vi "Test HRTF Computation.vi"() -> ()   [LabVIEW 2015]
uses:
  Typedefs/HRTF-Window.ctl
  Typedefs/HRTF-Window Type.ctl
  <vilib>/Analysis/2dsp.llb/Real FFT.vi
  <vilib>/Analysis/2dsp.llb/Inverse Real FFT.vi
  <vilib>/Analysis/2dsp.llb/Rational Resample (single channel, DBL).vi
  Utility VIs/Conversion VIs/Create Waveform Cluster (1D).vi
  <vilib>/Analysis/NI_AALPro.lvlib
panel:
  in  "Window":T1={"Type"=enum."Hanning", "Length (ms)"=6.0, "Center (ms)"=5.0}
  out "Waveform Graph":cluster{dbl, "dx":dbl, "Y":dbl[]}(graph)
  in  "Path":path=path "D:/Data/HRTF/E02/work/Ear-elev0-az-60_L.txt"
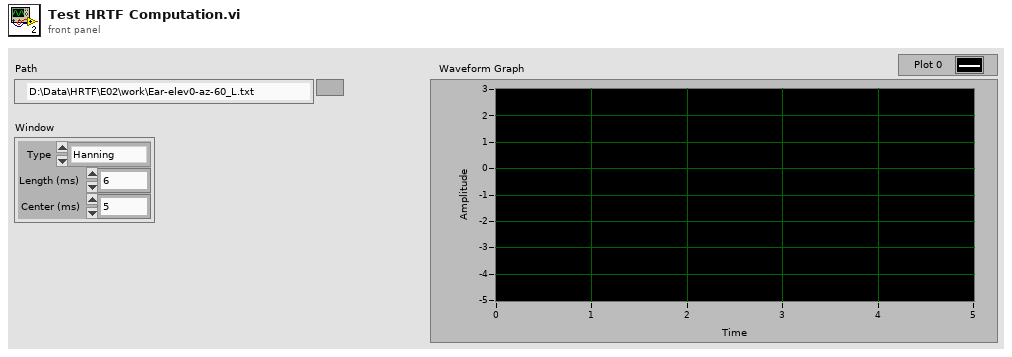
[diagram p1: front panel]
types:
  T1 = typedef "HRTF-Window.ctl" = cluster{"Type":T2, "Length (ms)":dbl, "Center (ms)":dbl}
  T2 = typedef "HRTF-Window Type.ctl" = enum16{"None", "Hanning"}
  T3 = typedef "HRTF-Parameters.ctl" = cluster{"Fs (Hz)":dbl, "atten (dB)":dbl, "Waveform":T4, "Freq Res (Hz)":dbl, "Order":i32, "Averages":i32, "seed":i64, "Window":T1}
  T4 = typedef "HRTF-Waveform.ctl" = enum16{"Chirp", "MLS"}
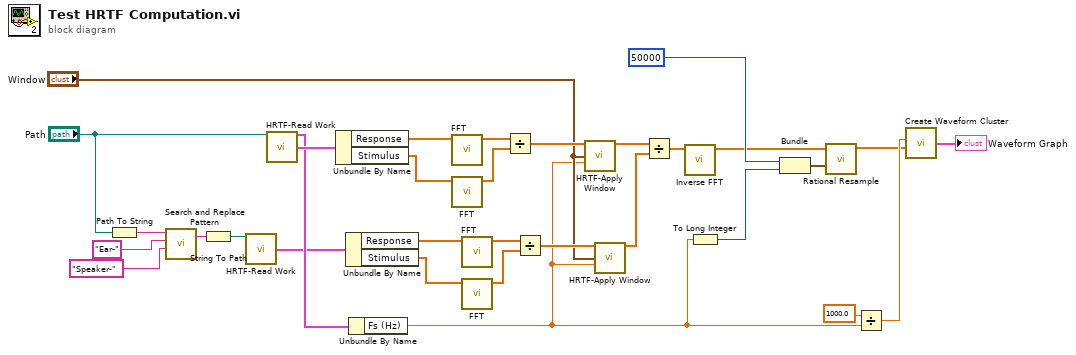
[diagram p0: block diagram]
diagram:
  n1 = Path To String(path="Path") -> (string=w21:string)
  n2 = call <vilib>:"Search and Replace Pattern.vi"("string"=w21, "regular expression (\"\")"="Ear-" ("regular expression (\"\")"), "replace string (\"\")"="Speaker-" ("regular expression (\"\")")) -> ("result string"=w18:string)  [unwired: 2 in, 1 out]
  n3 = String To Path(string=w18) -> (path=w17:path)
  n4 = call "HRTF-Read Work.vi"("path"=w17) -> ("Result"=w10:cluster{"Stimulus":dbl[], "Response":dbl[]})  [unwired: 12 in, 2 out]
  n5 = call "HRTF-Read Work.vi"("path"="Path") -> ("Params"=w29:T3, "Result"=w32:cluster{"Stimulus":dbl[], "Response":dbl[]})  [unwired: 12 in, 1 out]
  n6 = Unbundle By Name(w32) -> ("Response"=w25:dbl[], "Stimulus"=w31:dbl[])
  n7 = Unbundle By Name(w10) -> ("Response"=w14:dbl[], "Stimulus"=w16:dbl[])
  n8 = Unbundle By Name(w29) -> ("Fs (Hz)"=w6:dbl)
  n9 = call-poly <vilib>:"FFT.vi"("X"=w25) -> ("FFT {X}"=w24:cdb[])  [unwired: 9 in, 1 out]
  n10 = call-poly <vilib>:"FFT.vi"("X"=w31) -> ("FFT {X}"=w30:cdb[])  [unwired: 9 in, 1 out]
  n11 = call-poly <vilib>:"FFT.vi"("X"=w14) -> ("FFT {X}"=w13:cdb[])  [unwired: 9 in, 1 out]
  n12 = call-poly <vilib>:"FFT.vi"("X"=w16) -> ("FFT {X}"=w15:cdb[])  [unwired: 9 in, 1 out]
  n13 = Divide(x=w24, y=w30) -> (x/y=w23:cdb[])
  n14 = Divide(x=w13, y=w15) -> (x/y=w12:cdb[])
  n15 = call "HRTF-Apply Window.vi"("Array in"=w23, "Window"="Window", "Fs (Hz)"=w6) -> ("Array out"=w8:cdb[])  [unwired: 11 in, 1 out]
  n16 = call "HRTF-Apply Window.vi"("Array in"=w12, "Window"="Window", "Fs (Hz)"=w6) -> ("Array out"=w7:cdb[])  [unwired: 11 in, 1 out]
  n17 = Divide(x=w8, y=w7) -> (x/y=w9:cdb[])
  n18 = call-poly <vilib>:"Inverse FFT.vi"("FFT {X}"=w9) -> ("X"=w2:dbl[])  [unwired: 9 in, 1 out]
  n19 = To Long Integer(number=w6) -> (32bit integer=w5:i32)
  n20 = Bundle(50000, w5) -> (w3:cluster{i32, i32})  [unwired: 1 in]
  n21 = call-poly <vilib>:"Rational Resample.vi"("resample factor"=w3, "X"=w2) -> ("Y"=w1:dbl[])  [unwired: 7 in, 2 out]
  n22 = Divide(x=1000.0, y=w6) -> (x/y=w27:dbl)
  n23 = call-poly "Create Waveform Cluster.vi"("dx"=w27, "Y"=w1) -> ("waveform cluster"=→"Waveform Graph":cluster{dbl, "dx":dbl, "Y":dbl[]})  [unwired: 3 in]
